vi "User Interface.vi"(8 "error in (no error)":errorcluster, 9 "index":i32, 10 "User Interface Events":refnum<class "User Interface Events.lvclass">, 11 "Configuration in":refnum<class "Configuration.lvclass">) -> (0 "error out":errorcluster, 3 "Configuration out":refnum<class "Configuration.lvclass">)   [LabVIEW 2017, in "DSF Core.lvlib" / "Core Transfer User Interface.lvclass"]
uses:
  Core Transfer User Interface.lvclass
  Configuration/Configuration.lvclass
  User Interface Events/User Interface Events.lvclass
  Configuration/Core/Transfer/Core Transfers Configuration.lvclass
  C:/Git/DSF/Core/Classes/Configuration/Configuration.lvclass
panel:
  in  "Name":string
  out "Data Version":string
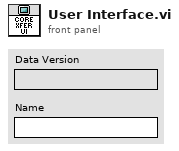
[diagram p1: front panel]
types:
  T1 = typedef "DSF Core.lvlib/DSF Core Transfer Configuration.ctl" = cluster{"name":string}
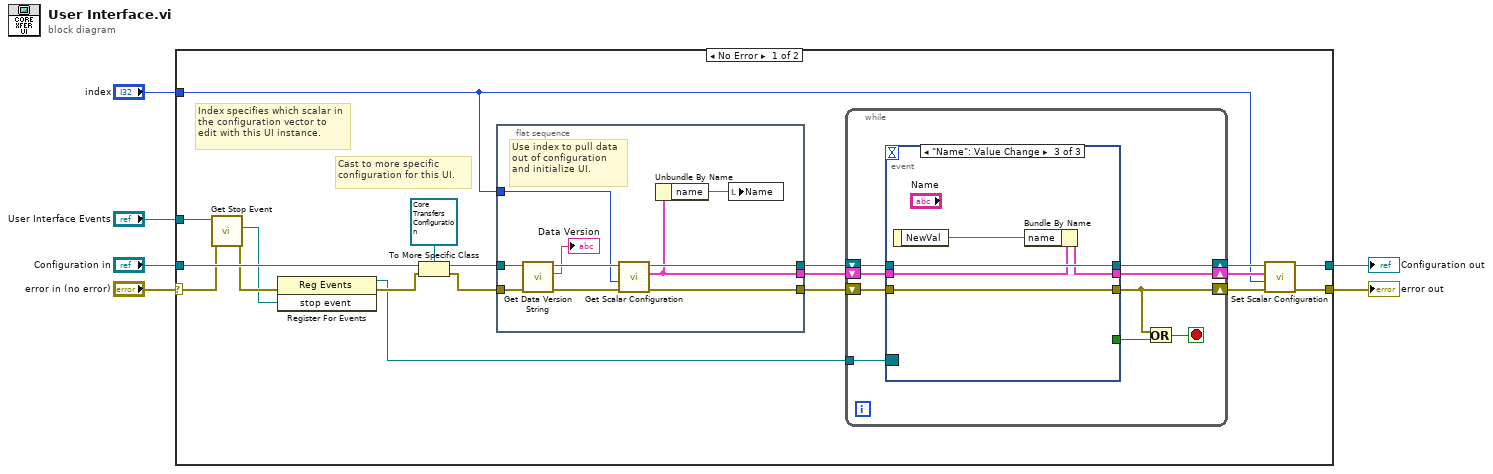
[diagram p0: block diagram]
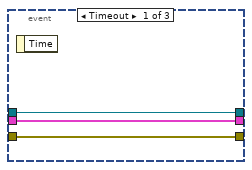
[diagram p2: hidden frame]
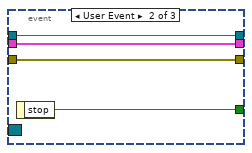
[diagram p3: hidden frame]
diagram:
  n1 = case shown="No Error" "error in (no error)" {
    selector: "error in (no error)" -> [w18 w58]
    tunnel: [w8 w58] -> w6
    tunnel: "index" -> [w7 _]
    tunnel: "Configuration in" -> [w21 w57]
    tunnel: [w9 w57] -> w2
    tunnel: "User Interface Events" -> [w19 _]
    frame No Error {
      # "Index specifies which scalar in the configuration vector to edit with this UI instance."
      # "Cast to more specific configuration for this UI."
      n2 = call "Get Stop Event.vi"("error in (no error)"=w18, "User Interface Events in"=w19) -> ("error out"=w17:errorcluster, "stop event"=w14:refnum<user-event>)  [unwired: 7 in, 1 out]
      n3 = register-events(error in=w17, w14) -> (reference out=w15:refnum<event-registration>, error out=w16:errorcluster)  [unwired: 1 in]
      n4 = To More Specific Class(target class=refnum<class "Core Transfers Configuration.lvclass"> refnum ("Configuration out"), reference=w21, error in=w16) -> (specific class reference=w25:refnum<class "Core Transfers Configuration.lvclass">, error out=w20:errorcluster)
      n5 = flat-sequence {
        tunnel: [w30] -> w22
        tunnel: w20 -> [w35]
        tunnel: w25 -> [w34]
        tunnel: [w31] -> w23
        tunnel: w7 -> [w28]
        tunnel: [w27] -> w13
        frame #0 {
          # "Use index to pull data out of configuration and initialize UI."
          n6 = call "Get Data Version String.vi"("error in (no error)"=w35, "Configuration in"=w34) -> ("error out"=w33:errorcluster, "data version"=→"Data Version":string, "Configuration out"=w32:refnum<class "Core Transfers Configuration.lvclass">)  [unwired: 7 in]
          n7 = call "Get Scalar Configuration.vi"("error in (no error)"=w33, "index"=w28, "Core Transfers Configuration in"=w32) -> ("error out"=w30:errorcluster, "transfer configuration"=w27:T1, "Core Transfers Configuration out"=w31:refnum<class "Core Transfers Configuration.lvclass">)  [unwired: 6 in]
          n8 = Unbundle By Name(w27) -> ("name"=w26:string)
          n9 = local write "Name"(w26) -> ()
        }
      }
      n10 = while {
        tunnel: w15 -> [w44]
        shift-right: [w42] -> w12
        shift-left: w22 -> [w43]
        shift-right: [w38] -> w11
        shift-left: w23 -> [w39]
        shift-right: [w36] -> w10
        shift-left: w13 -> [w37]
        stop <- w41 stop-if-true
        n11 = event shown="[2] \"Name\": Value Change" {
          selector: w44 -> [_ _ _]
          dyn-events: _ -> [_ _ _]
          timeout: _ -> [_ _ _]
          tunnel: [_ w49 _] -> w40
          tunnel: w43 -> [w47 w51 w56]
          tunnel: [w47 w51 w56] -> w42
          tunnel: w39 -> [w46 w50 w55]
          tunnel: [w46 w50 w55] -> w38
          tunnel: w37 -> [w45 w48 w52]
          tunnel: [w45 w48 w54] -> w36
          event Timeout {
            n12 = event-data() -> ()  [unwired: 1 in, 1 out]
          }
          event User Event {
            n13 = event-data() -> ("stop"=w49:bool)  [unwired: 1 in]
          }
          event "Name": Value Change {
            n14 = event-data() -> ("NewVal"=w53:string)  [unwired: 1 in]
            n15 = Bundle By Name(cluster=w52, "name"=w53) -> (w54:T1)
          }
        }
        n16 = Or(x=w42, y=w40) -> (x .or. y?=w41:bool)
      }
      n17 = call "Set Scalar Configuration.vi"("error in (no error)"=w12, "index"=w7, "transfer configuration"=w10, "Core Transfers Configuration in"=w11) -> ("error out"=w8:errorcluster, "Core Transfers Configuration out"=w9:refnum<class "Core Transfers Configuration.lvclass">)  [unwired: 6 in]
    }
    frame Error {
    }
  }
  "error out" <- w6
  "Configuration out" <- w2
